vi "DB_Lee_IP_equipos.vi"() -> (0 "error out":errorcluster, 2 "IP_EQUIPO":string[](array[string]))   [LabVIEW 2018]
uses:
  <vilib>/addons/database/Connection.llb/DB Tools Open Connec (Path).vi
  <vilib>/addons/database/Connection.llb/Conn Execute.vi
  <vilib>/addons/database/Recordset.llb/Rec Fetch Recordset Data (R).vi
  <vilib>/addons/database/Recordset.llb/Rec Destroy - Connection.vi
  <vilib>/addons/database/_DB Variant To Data/Database Variant To Data.xnode
  <vilib>/addons/database/NI_Database_API.lvlib
panel:
  in  "error in (no error)":errorcluster
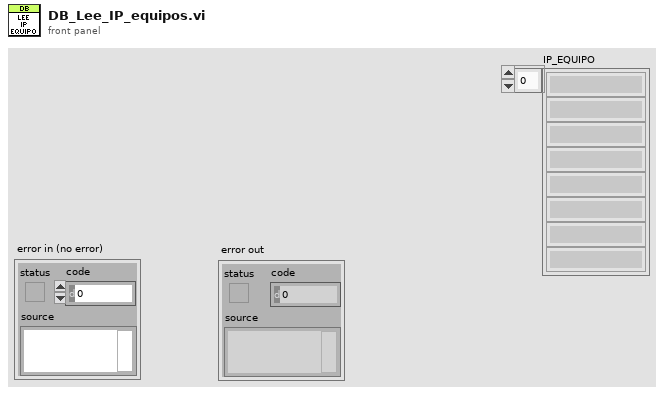
[diagram p1: front panel]
types:
  T1 = typedef "NI_Database_API.lvlib/Conn ObjectReference.ctl" = refnum<k1>
  T2 = typedef "NI_Database_API.lvlib/Rec ObjectReference.ctl" = refnum<k1>
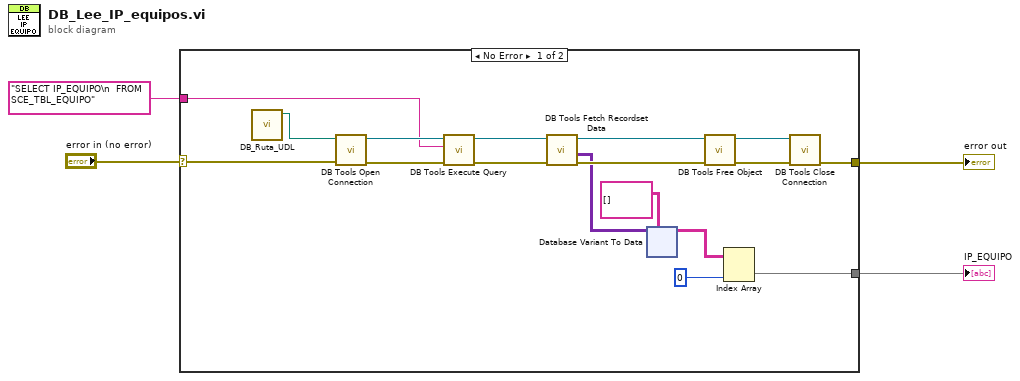
[diagram p0: block diagram]
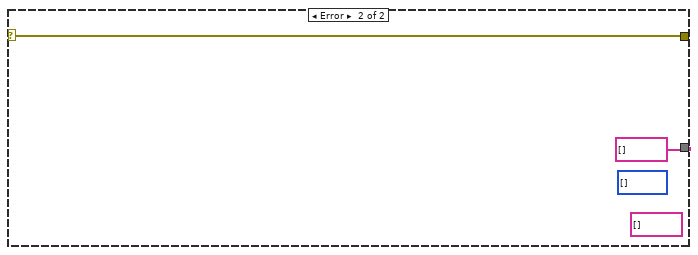
[diagram p2: hidden frame]
diagram:
  n1 = case shown="No Error" "error in (no error)" {
    selector: "error in (no error)" -> [w16 w67]
    tunnel: [w18 w67] -> w4
    tunnel: "SELECT IP_EQUIPO\n  FROM SCE_TBL_EQUIPO" ("SQL") -> [w15 _]
    tunnel: [w11 string[] [] ("data")] -> w1
    frame No Error {
      n2 = call "DB_Ruta_UDL.vi"() -> ("UDL ruta"=w10:path)  [unwired: 11 in]
      n3 = call-poly <vilib>:"DB Tools Open Connection.vi"("error in (no error)"=w16, "connection information"=w10) -> ("error out"=w21:errorcluster, "connection reference"=w19:T1)  [unwired: 6 in]
      n4 = call-poly <vilib>:"DB Tools Execute Query.vi"("error in (no error)"=w21, "SQL query"=w15, "connection reference"=w19) -> ("error out"=w17:errorcluster, "recordset reference"=w14:T2)  [unwired: 5 in]
      n5 = call-poly <vilib>:"DB Tools Fetch Recordset Data.vi"("error in (no error)"=w17, "recordset reference"=w14) -> ("error out"=w12:errorcluster, "recordset data"=w7:variant[][], "recordset reference out"=w13:T2)  [unwired: 3 in]
      n6 = xnode "Database Variant To Data"("database variant"=w7, "type"=string[][] []) -> ("data"=w6:string[][])  [unwired: 1 in, 1 out]
      n7 = call-poly <vilib>:"DB Tools Free Object.vi"("error in (no error)"=w12, "recordset reference"=w13) -> ("error out"=w20:errorcluster, "connection reference"=w9:T1)  [unwired: 8 in]
      n8 = Index Array(array=w6, index (col)=0 ("disabled index (col)")) -> (element=w11:string[])  [unwired: 1 in]
      n9 = call <vilib>:"DB Tools Close Connection.vi"("error in (no error)"=w20, "connection reference"=w9) -> ("error out"=w18:errorcluster)  [unwired: 5 in]
    }
    frame Error {
      (unwired) string[] [] ("data")
      (unwired) i32[] []
    }
  }
  "error out" <- w4
  "IP_EQUIPO" <- w1
